vi "VerifyExperiment.vi"(11 "Experiment":T1={"File Path"=path "", "Operator"="", "Project"="", "Target Dose (dpa)"=0.0, "Sample"={"Name"="", "Description"="", "Molar Mass (g/mol)"=0.0, "Density (g/cm^3)"=0.0, "Irradiation Area (cm^2)"=0.0, "SRIM Damage Peak (disp * ions/cm)"=0.0}, "Beam Line"={"Type"=enum."Ion Beam Analysis", "Ion"=enum."H", "Charge State"=0, "Total Source Ion Energy (kV)"=nan}, "Runs"=[]} {"Beam Line"."Charge State" min=1}) -> (0 "Error Out":errorcluster, 3 "Experiment Valid?":bool)   [LabVIEW 2012]
uses:
  Experiment.ctl
  Sample.ctl
  BeamLine.ctl
  BeamLineType.ctl
  BeamLineIon.ctl
  ExperimentRun.ctl
  ExperimentRunTiming.ctl
  ExperimentRunDose.ctl
  ExperimentRunFluence.ctl
  ExperimentRunTotalCharge.ctl
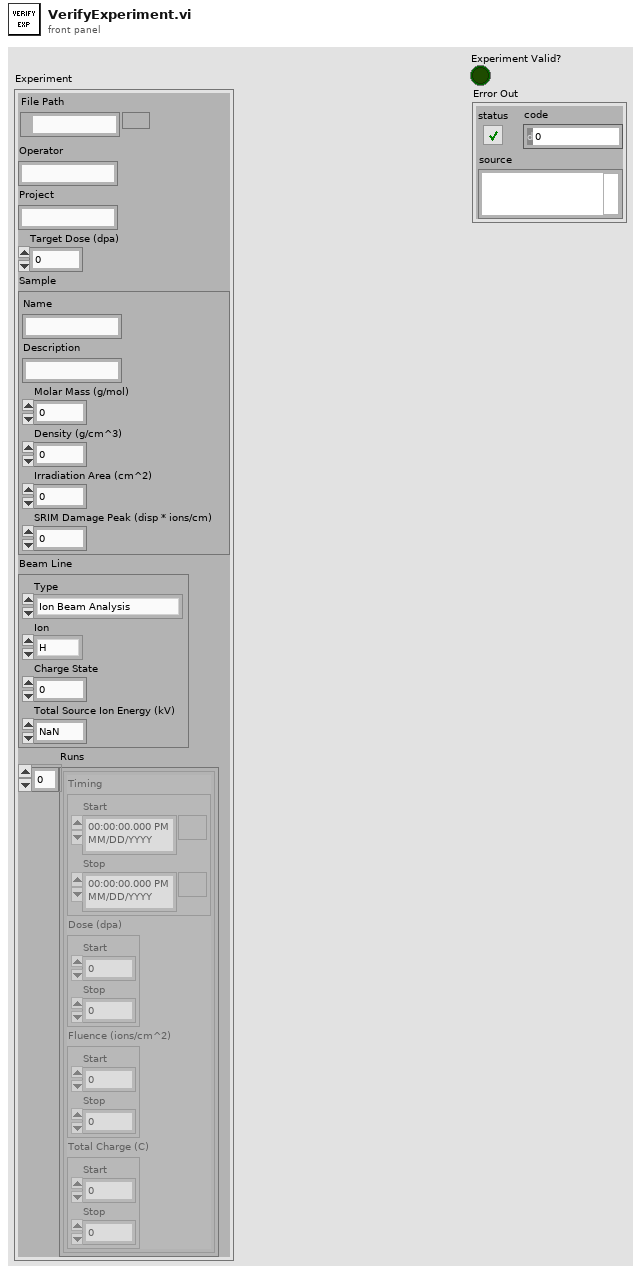
[diagram p1: front panel]
types:
  T1 = typedef "Experiment.ctl" = cluster{"File Path":path, "Operator":string, "Project":string, "Target Dose (dpa)":dbl, "Sample":T2, "Beam Line":T3, "Runs":T6[]}
  T2 = typedef "Sample.ctl" = cluster{"Name":string, "Description":string, "Molar Mass (g/mol)":dbl, "Density (g/cm^3)":dbl, "Irradiation Area (cm^2)":dbl, "SRIM Damage Peak (disp * ions/cm)":dbl}
  T3 = typedef "BeamLine.ctl" = cluster{"Type":T4, "Ion":T5, "Charge State":u8, "Total Source Ion Energy (kV)":dbl}
  T4 = typedef "BeamLineType.ctl" = enum16{"Ion Beam Analysis", "Auxiliary", "Radiation Damage"}
  T5 = typedef "BeamLineIon.ctl" = enum16{"H", "He", "C", "Fe", "Ni", "Pt", "Si", "Ag", "Au"}
  T6 = typedef "ExperimentRun.ctl" = cluster{"Timing":T7, "Dose (dpa)":T8, "Fluence (ions/cm^2)":T9, "Total Charge (C)":T10}
  T7 = typedef "ExperimentRunTiming.ctl" = cluster{"Start":timestamp, "Stop":timestamp}
  T8 = typedef "ExperimentRunDose.ctl" = cluster{"Start":dbl, "Stop":dbl}
  T9 = typedef "ExperimentRunFluence.ctl" = cluster{"Start":dbl, "Stop":dbl}
  T10 = typedef "ExperimentRunTotalCharge.ctl" = cluster{"Start":dbl, "Stop":dbl}
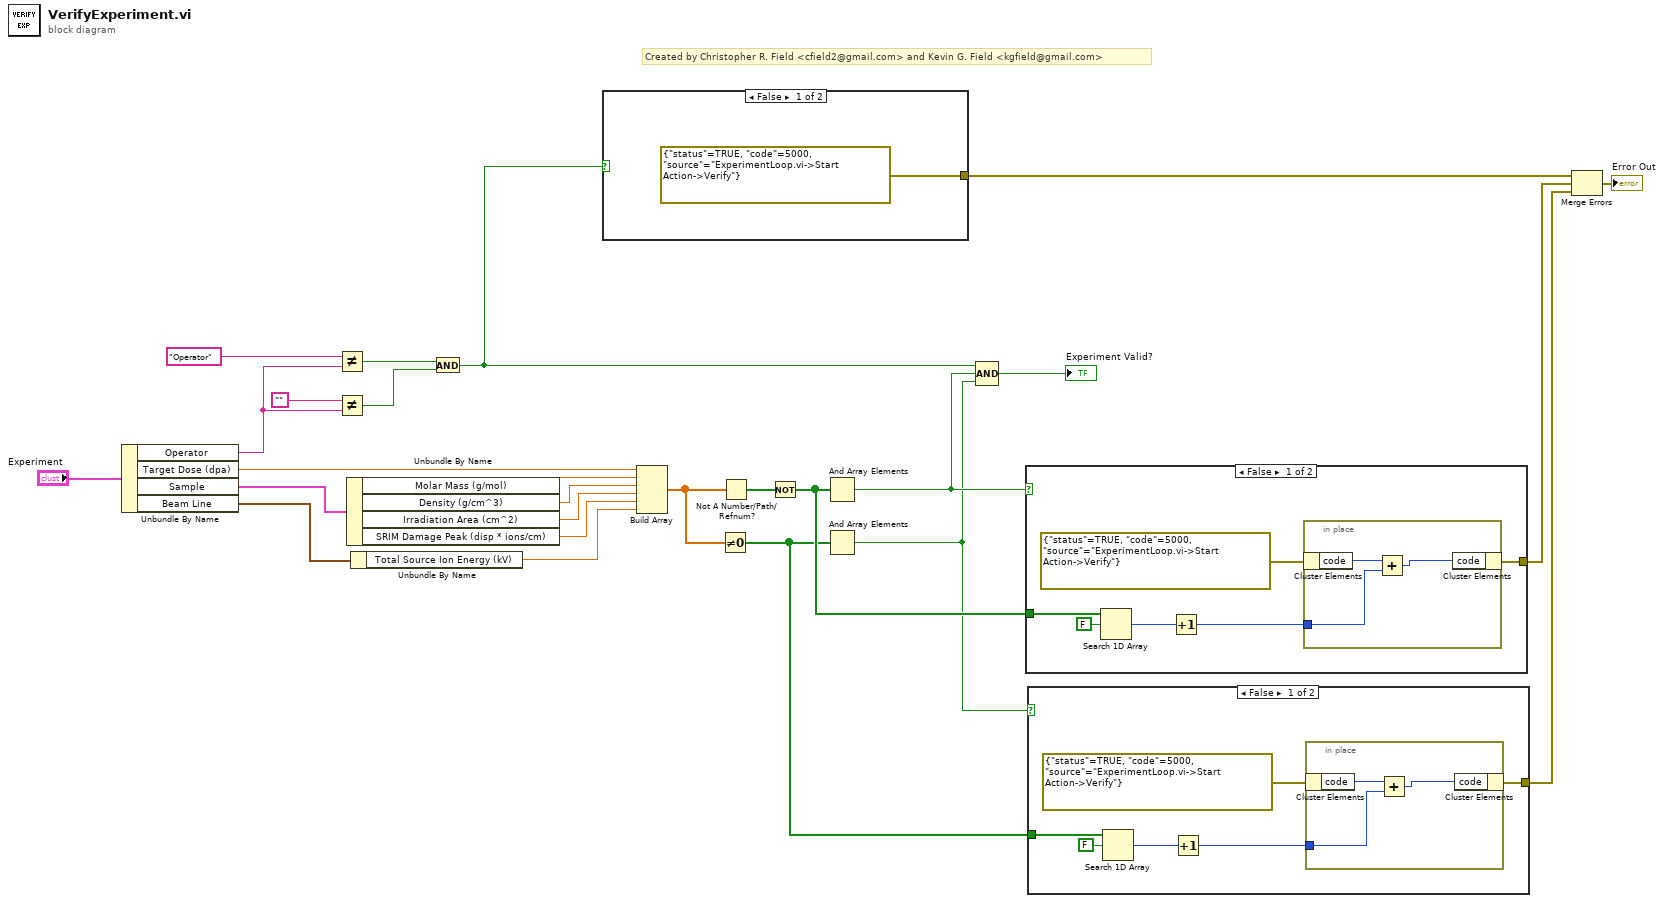
[diagram p0: block diagram]
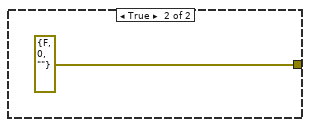
[diagram p2: hidden frame]
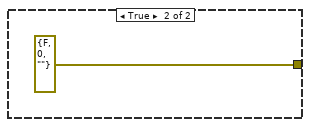
[diagram p3: hidden frame]
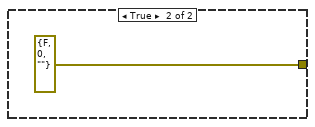
[diagram p4: hidden frame]
diagram:
  # "Created by Christopher R. Field <cfield2@gmail.com> and Kevin G. Field <kgfield@gmail.com>"
  n1 = Unbundle By Name("Experiment") -> ("Operator"=w14:string, "Target Dose (dpa)"=w18:dbl, "Sample"=w25:T2, "Beam Line"=w20:T3)
  n2 = Not Equal?(x="Operator", y=w14) -> (x != y?=w12:bool)
  n3 = Not Equal?(x="", y=w14) -> (x != y?=w11:bool)
  n4 = Unbundle By Name(w25) -> ("Molar Mass (g/mol)"=w24:dbl, "Density (g/cm^3)"=w23:dbl, "Irradiation Area (cm^2)"=w22:dbl, "SRIM Damage Peak (disp * ions/cm)"=w21:dbl)
  n5 = Unbundle By Name(w20) -> ("Total Source Ion Energy (kV)"=w19:dbl)
  n6 = And(x=w12, y=w11) -> (x .and. y?=w9:bool)
  n7 = case shown="False" w9 {
    tunnel: [errorcluster {"status"=TRUE, "code"=5000, "source"="ExperimentLoop.vi->Start Action->Verify"} ("error constant") errorcluster {"status"=FALSE, "code"=0, "source"=""} ("error constant")] -> w8
    frame False {
    }
    frame True {
    }
  }
  n8 = Build Array(w18, w24, w23, w22, w21, w19) -> (w16:dbl[])
  n9 = Not Equal To 0?(x=w16) -> (x != 0?=w3:bool[])
  n10 = Not A Number/Path/Refnum?(number/path/refnum=w16) -> (NaN/Path/Refnum?=w17:bool[])
  n11 = Not(x=w17) -> (.not. x?=w6:bool[])
  n12 = And Array Elements(Boolean array=w6) -> (logical AND=w7:bool)
  n13 = And Array Elements(Boolean array=w3) -> (logical AND=w4:bool)
  n14 = Compound Arithmetic op=AND(w9, w7, w4) -> (→"Experiment Valid?":bool)
  n15 = case shown="False" w7 {
    tunnel: w6 -> [w34 _]
    tunnel: [w29 errorcluster {"status"=FALSE, "code"=0, "source"=""} ("error constant")] -> w5
    frame False {
      n16 = Search 1D Array(1D array=w34, element=FALSE) -> (index of element=w31:i32)  [unwired: 1 in]
      n17 = Increment(x=w31) -> (x+1=w30:i32)
      n18 = in-place {
        in-place-border: w30 -> [w36]
        n19 = in-place-cluster #1(errorcluster {"status"=TRUE, "code"=5000, "source"="ExperimentLoop.vi->Start Action->Verify"} ("error constant")) -> ("code"=w37:i32)
        n20 = Add(x=w37, y=w36) -> (x+y=w35:i32)
        n21 = in-place-cluster #1("code"=w35) -> (w29:errorcluster)
      }
    }
    frame True {
    }
  }
  n22 = case shown="False" w4 {
    tunnel: w3 -> [w44 _]
    tunnel: [w39 errorcluster {"status"=FALSE, "code"=0, "source"=""} ("error constant")] -> w2
    frame False {
      n23 = Search 1D Array(1D array=w44, element=FALSE) -> (index of element=w41:i32)  [unwired: 1 in]
      n24 = Increment(x=w41) -> (x+1=w40:i32)
      n25 = in-place {
        in-place-border: w40 -> [w46]
        n26 = in-place-cluster #2(errorcluster {"status"=TRUE, "code"=5000, "source"="ExperimentLoop.vi->Start Action->Verify"} ("error constant")) -> ("code"=w47:i32)
        n27 = Add(x=w47, y=w46) -> (x+y=w45:i32)
        n28 = in-place-cluster #2("code"=w45) -> (w39:errorcluster)
      }
    }
    frame True {
    }
  }
  n29 = Merge Errors(w8, w5, w2) -> (→"Error Out":errorcluster)
